vi "Error.vi"(6 "Abort if errors":bool, 8 "error in (no error)":errorcluster, 10 "Error":errorcluster, 11 "Process Events":T1) -> (0 "error out":errorcluster, 3 "Process Events out":T1)   [LabVIEW 2015]
uses:
  Process Events.ctl
  Simple Progress Bar.lvlib
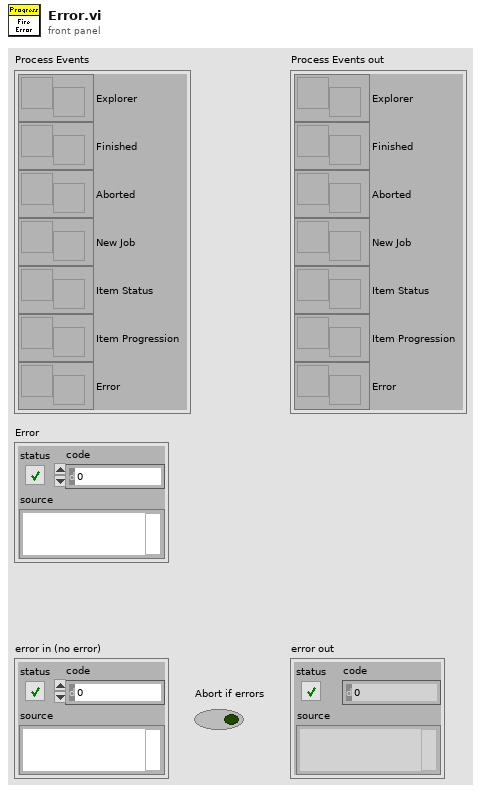
[diagram p1: front panel]
types:
  T1 = typedef "Simple Progress Bar.lvlib/Process Events.ctl" = cluster{"Explorer":refnum<user-event>, "Finished":refnum<user-event>, "Aborted":refnum<user-event>, "New Job":refnum<user-event>, "Item Status":refnum<user-event>, "Item Progression":refnum<user-event>, "Error":refnum<user-event>}
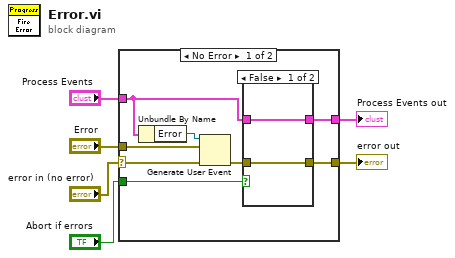
[diagram p0: block diagram]
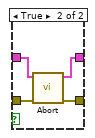
[diagram p2: hidden frame]
diagram:
  n1 = case shown="No Error" "error in (no error)" {
    selector: "error in (no error)" -> [w13 w21]
    tunnel: "Process Events" -> [w11 w22]
    tunnel: [w7 w22] -> w4
    tunnel: [w8 w21] -> w3
    tunnel: "Error" -> [w12 _]
    tunnel: "Abort if errors" -> [w9 _]
    frame No Error {
      n2 = Unbundle By Name(w11) -> ("Error"=w14:refnum<user-event>)
      n3 = Generate User Event(user event=w14, event data cluster=w12, error in=w13) -> (error out=w10:errorcluster)  [unwired: 1 in, 1 out]
      n4 = case shown="False" w9 {
        tunnel: w11 -> [w16 w17]
        tunnel: w10 -> [w15 w20]
        tunnel: [w15 w19] -> w8
        tunnel: [w16 w18] -> w7
        frame False {
        }
        frame True {
          n5 = call "Abort.vi"("error in (no error)"=w20, "Process Events"=w17) -> ("error out"=w19:errorcluster, "Process Events out"=w18:T1)  [unwired: 8 in]
        }
      }
    }
    frame Error {
    }
  }
  "error out" <- w3
  "Process Events out" <- w4
